vi "5.2.vi"() -> ()   [LabVIEW 2017]
panel:
  out "布尔":bool
  in  "簇":cluster{"姓名":string, "是否注册":bool, "学号":dbl}
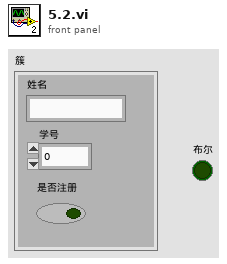
[diagram p1: front panel]
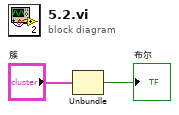
[diagram p0: block diagram]
diagram:
  n1 = Unbundle("簇") -> ("是否注册"=→"布尔":bool)  [unwired: 2 out]
